vi "Configure Limit Test Template.vi"(6 "Destination Reference (0:Reference Waveform 1)":i32(ring) items=["Reference Waveform 1", "Reference Waveform 2", "Reference Waveform 3", "Reference Waveform 4"], 7 "Horizontal (0.0 mdiv)":dbl, 8 "error in (no error)":errorcluster, 9 "Vertical (0.0 mdiv)":dbl, 10 "Source (0:Channel 1)":i32(ring) items=["Channel 1", "Channel 2", "Channel 3", "Channel 4", "Math"], 11 "VISA resource name":refnum<visa-resource-name>) -> (0 "error out":errorcluster, 3 "VISA resource name out":refnum<visa-resource-name>)   [LabVIEW 2012, in "Tektronix TDS 200 1000 2000 Series.lvlib"]
doc: "This VI configures the settings for a limit test single template.\n\n<b>Note(s):</b>\nThis VI does not check the instrument status."
uses:
  <instrlib>/Tektronix TDS 200 1000 2000 Series/Tektronix TDS 200 1000 2000 Series.lvlib
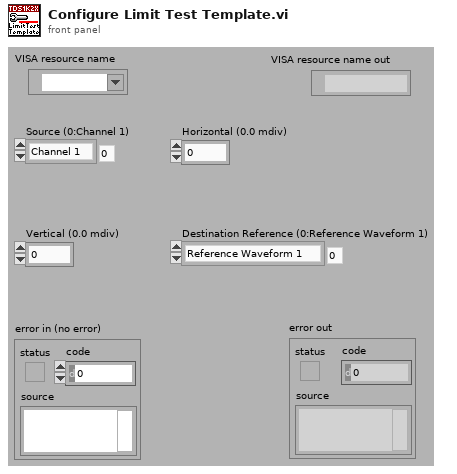
[diagram p1: front panel]
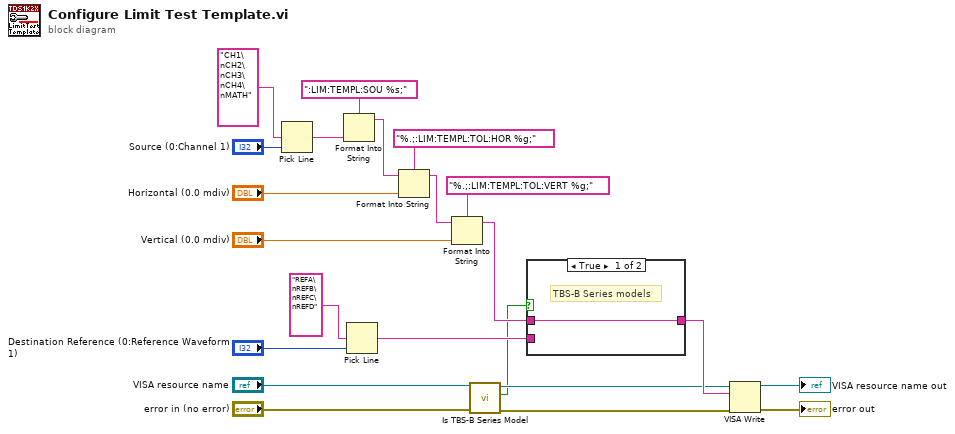
[diagram p0: block diagram]
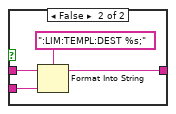
[diagram p2: hidden frame]
diagram:
  n1 = Pick Line(multi-line string="CH1\nCH2\nCH3\nCH4\nMATH", line index="Source (0:Channel 1)") -> (output string=w18:string)  [unwired: 1 out]
  n2 = Format Into String(format string=":LIM:TEMPL:SOU %s;", w18) -> (resulting string=w17:string)  [unwired: 2 in, 1 out]
  n3 = Pick Line(multi-line string="REFA\nREFB\nREFC\nREFD", line index="Destination Reference (0:Reference Waveform 1)") -> (output string=w13:string)  [unwired: 1 out]
  n4 = Format Into String(format string="%.;:LIM:TEMPL:TOL:HOR %g;", initial string=w17, "Horizontal (0.0 mdiv)") -> (resulting string=w15:string)  [unwired: 1 in, 1 out]
  n5 = Format Into String(format string="%.;:LIM:TEMPL:TOL:VERT %g;", initial string=w15, "Vertical (0.0 mdiv)") -> (resulting string=w12:string)  [unwired: 1 in, 1 out]
  n6 = call <instrlib>:"Is TBS-B Series Model.vi"("error in (no error)"="error in (no error)", "VISA resource name"="VISA resource name") -> ("error out"=w2:errorcluster, "Is TBS-B Series Model"=w1:bool, "VISA resource name out"=w3:refnum<visa-resource-name>)  [unwired: 7 out]
  n7 = case shown="True" w1 {
    tunnel: w13 -> [_ w26]
    tunnel: w12 -> [w23 w25]
    tunnel: [w23 w24] -> w11
    frame True {
      # "TBS-B Series models"
    }
    frame False {
      n8 = Format Into String(format string=":LIM:TEMPL:DEST %s;", initial string=w25, w26) -> (resulting string=w24:string)  [unwired: 1 in, 1 out]
    }
  }
  n9 = VISA Write(VISA resource name=w3, write buffer=w11, error in (no error)=w2) -> (VISA resource name out=→"VISA resource name out":refnum<visa-resource-name>, error out=→"error out":errorcluster)  [unwired: 1 out]
